vi "CheckExplicit.vi"(8 "error in (no error)":errorcluster, 11 "PathTokenizer in":refnum<class "PathTokenizer.lvclass">) -> (0 "error out":errorcluster, 3 "PathTokenizer out":refnum<class "PathTokenizer.lvclass">)   [LabVIEW 2019, in "PathTokenizer.lvclass"]
uses:
  PathTokenizer.lvclass
  PathTokenizer.lvclass/PathTokenizer.ctl
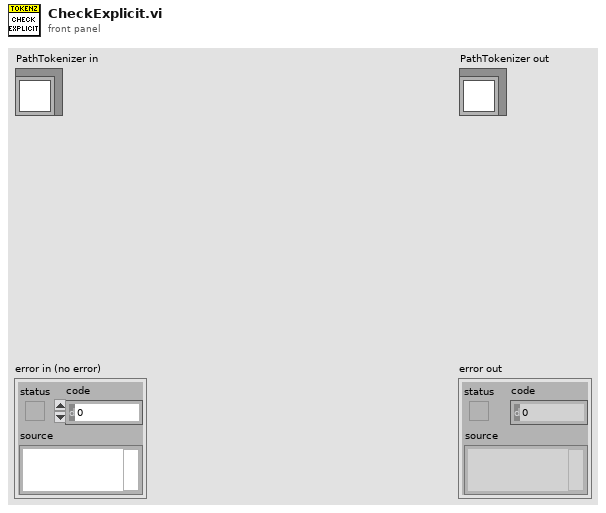
[diagram p1: front panel]
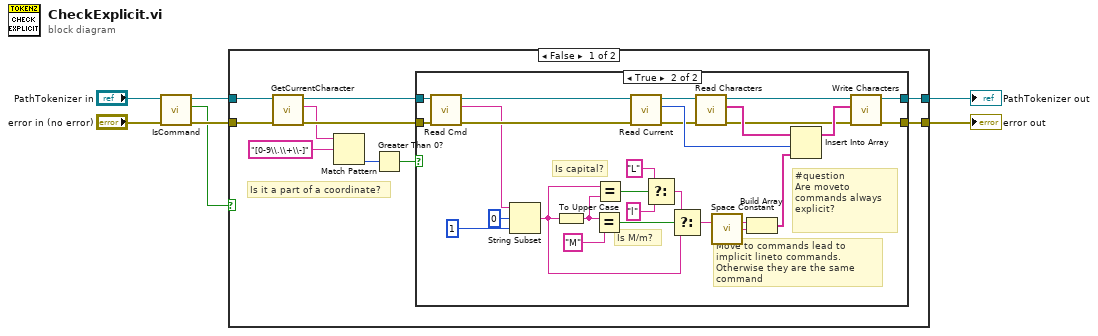
[diagram p0: block diagram]
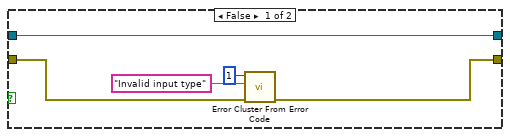
[diagram p2: hidden frame]
diagram:
  n1 = call "IsCommand.vi"("error in (no error)"="error in (no error)", "PathTokenizer in"="PathTokenizer in") -> ("error out"=w3:errorcluster, "Is Command"=w1:bool, "PathTokenizer out"=w5:refnum<class "PathTokenizer.lvclass">)  [unwired: 7 in]
  n2 = case shown="False" w1 {
    tunnel: w5 -> [w12 w51]
    tunnel: [w17 w51] -> w4
    tunnel: w3 -> [w11 w50]
    tunnel: [w16 w50] -> w2
    frame False {
      # "Is it a part of a coordinate?"
      n3 = call "GetCurrentCharacter.vi"("error in (no error)"=w11, "PathTokenizer in"=w12) -> ("error out"=w9:errorcluster, "Current Character"=w8:string, "PathTokenizer out"=w10:refnum<class "PathTokenizer.lvclass">)  [unwired: 7 in]
      n4 = Match Pattern(string=w8, regular expression="[0-9\\.\\+\\-]") -> (offset past match=w14:i32)  [unwired: 1 in, 3 out]
      n5 = Greater Than 0?(x=w14) -> (x > 0?=w13:bool)
      n6 = case shown="True" w13 {
        tunnel: [w22 w49] -> w17
        tunnel: w10 -> [w22 w27]
        tunnel: [w21 w28] -> w16
        tunnel: w9 -> [w18 w26]
        frame False {
          n7 = call <vilib>:"Error Cluster From Error Code.vi"("error in (no error)"=w18, "error message (\"\")"="Invalid input type" ("error message (\"\")"), "error code (0)"=1) -> ("error out"=w21:errorcluster)  [unwired: 6 in]
        }
        frame True {
          # "#question\nAre moveto commands always explicit?"
          # "Move to commands lead to implicit lineto commands. Otherwise they are the same command"
          # "Is M/m?"
          # "Is capital?"
          n8 = call "Read Cmd.vi"("error in (no error)"=w26, "PathTokenizer in"=w27) -> ("error out"=w24:errorcluster, "Cmd"=w23:string, "PathTokenizer out"=w25:refnum<class "PathTokenizer.lvclass">)  [unwired: 7 in]
          n9 = String Subset(string=w23, offset (0)=0, length (rest)=1 ("length (rest)")) -> (substring=w44:string)
          n10 = To Upper Case(1:w44) -> (0:w43:string)
          n11 = Equal?(x=w43, y="M") -> (x = y?=w46:bool)
          n12 = Equal?(x=w44, y=w43) -> (x = y?=w42:bool)
          n13 = call "Read Current.vi"("error in (no error)"=w24, "PathTokenizer in"=w25) -> ("error out"=w30:errorcluster, "Current"=w35:i32, "PathTokenizer out"=w38:refnum<class "PathTokenizer.lvclass">)  [unwired: 7 in]
          n14 = Select(t="L", s=w42, f="l") -> (s? t:f=w39:string)
          n15 = Select(t=w39, s=w46, f=w44) -> (s? t:f=w33:string)
          n16 = call "Read Characters.vi"("error in (no error)"=w30, "PathTokenizer in"=w38) -> ("error out"=w29:errorcluster, "Characters"=w37:string[], "PathTokenizer out"=w34:refnum<class "PathTokenizer.lvclass">)  [unwired: 7 in]
          n17 = call <vilib>:"Space Constant.vi"() -> ("String"=w32:string)
          n18 = Build Array(w33, w32) -> (w31:string[])
          n19 = Insert Into Array(array=w37, index=w35, new element=w31) -> (w36:string[])
          n20 = call "Write Characters.vi"("error in (no error)"=w29, "Characters"=w36, "PathTokenizer in"=w34) -> ("error out"=w28:errorcluster, "PathTokenizer out"=w49:refnum<class "PathTokenizer.lvclass">)  [unwired: 7 in]
        }
      }
    }
    frame True {
    }
  }
  "error out" <- w2
  "PathTokenizer out" <- w4
